vi "fpga_Fund FIFO Control.vi"(0 "Time stamp":fxp<+,64,32> format="%.42g", 1 "reset":bool, 2 "nominal frequency":enum16{"50 Hz", "60 Hz"}(ring), 5 "Frequency":fxp<+,32,8>, 7 "#ch":fxp<+,5,5>, 9 "PMU VI input valid":bool, 11 "PMU VI output valid":bool) -> (4 "Time Stamp out":fxp<+,64,32> format="%.42g", 8 "output frequency":T1 {"frequency timestamp [s]" format="%#.6g"})   [LabVIEW 2012, in "NI_EP_Protection_FPGA.lvlib"]
uses:
  <vilib>/addons/Electrical Power/Protection/NI_EP_Protection_FPGA.lvlib
  <vilib>/addons/Electrical Power/Protection/Protection Measurement/subVIs/fpga_OutputFrequency.ctl
  <vilib>/rvi/DataTransferAndStorage/Container/Common/niFpgaContainerMetaDataKey.ctl
  <vilib>/rvi/DataTransferAndStorage/Container/Common/niFpgaContainerState.ctl
  <vilib>/rvi/DataTransferAndStorage/Container/Common/niFpgaDataTypeControl.ctl
  <vilib>/rvi/DataTransferAndStorage/Container/Common/niFpgaContainerImplementationControl.ctl
  <vilib>/rvi/DataTransferAndStorage/Container/Common/niFpgaContainerArbitrationOptionsControl.ctl
  <vilib>/rvi/DataTransferAndStorage/Container/Common/niFpgaTransferTypeControl.ctl
  <vilib>/rvi/DataTransferAndStorage/Container/Common/niFpgaContainerInitializationParameters.ctl
  <vilib>/rvi/Memory/Memory_Types/niFpgaMemoryInterfaceConfiguration.ctl
  <vilib>/rvi/FIFO/Fifo_Types/niFpgaFifoControlLogicControl.ctl
  <vilib>/rvi/DataTransferAndStorage/Container/Common/niFpgaContainerGetUniqueNameForEmu.vi
  <vilib>/rvi/DataTransferAndStorage/Container/Common/niFpgaContainerSetEmuInfo.vi
  <vilib>/rvi/eio/common/nirviEmuReportErrorAndStop.vi
  <vilib>/rvi/Emulation/niFpgaSctlEmulationGetInTimedLoop.vi
  <vilib>/rvi/FIFO/Fifo_Resource/nirvififoEmulationSetSize.vi
  <vilib>/rvi/Emulation/niFpgaSctlEmulationFifoFullMgr.vi
  <vilib>/rvi/errors/niFpgaSetErrorForExecOnDevCompSimple.vi
  <vilib>/rvi/Emulation/niFpgaSctlEmulationResourceMgr.vi
  <vilib>/rvi/LocalResourceManager/LocalResourceManager.xnode
  <vilib>/rvi/DataTransferAndStorage/Container/XNode/niFpgaContainer.xnode
  <vilib>/rvi/FIFO/Fifo_Resource/nirvififoEmulationRead.vi
  <vilib>/rvi/FXPMathLib/basic elements/FxpDiscreteDelay/XNode/nifxpmath_DiscreteDelay.xnode
  <vilib>/rvi/FXPMathLib/FxpSub/XNode/nifxpmath_Sub.xnode
  <vilib>/rvi/FIFO/Fifo_Resource/nirvififoEmulationWrite.vi
  <vilib>/addons/Electrical Power/PQ/Resampling/NI_EP_Resample_FPGA.lvlib
  <vilib>/rvi/FXPMathLib/sim/FxpSim.dll
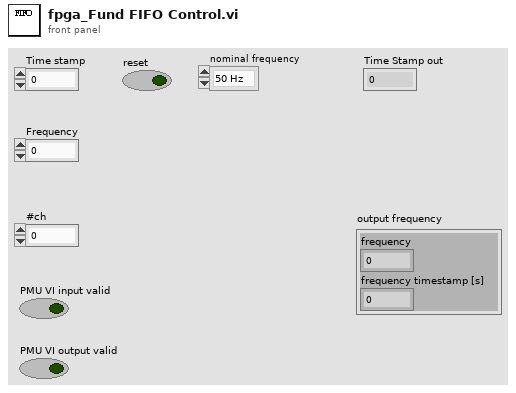
[diagram p1: front panel]
types:
  T1 = typedef "NI_EP_Protection_FPGA.lvlib/fpga_OutputFrequency.ctl" = cluster{"frequency":fxp<+,32,8>, "frequency timestamp [s]":fxp<+,64,32>}
  T2 = cluster{"frequency":fxp<+,32,8>, "frequency timestamp [s]":fxp<+,64,32>}
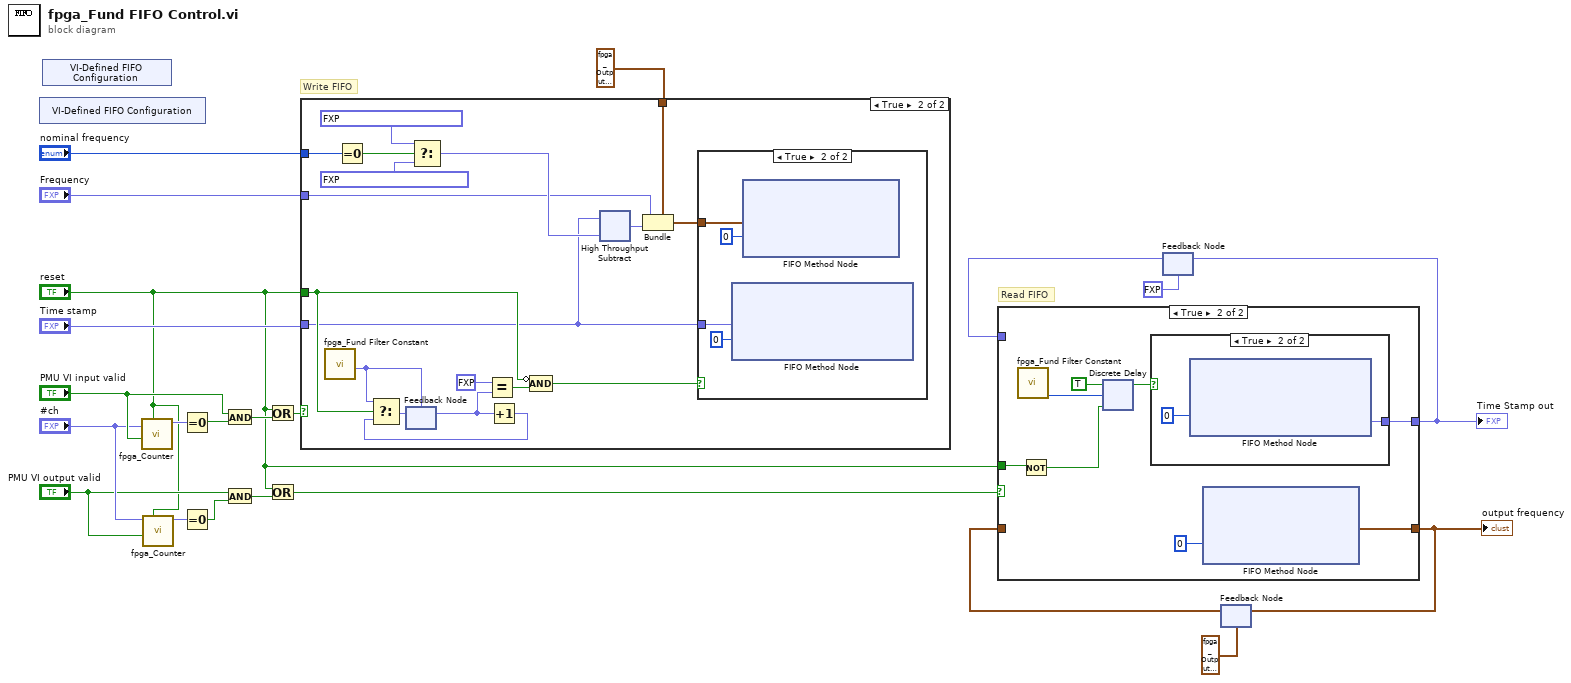
[diagram p0: block diagram]
diagram:
  # "Read FIFO"
  # "Write FIFO"
  n1 = xnode "VI-Defined FIFO Configuration"() -> ()  [unwired: 1 out]
  n2 = xnode "VI-Defined FIFO Configuration"() -> ()  [unwired: 1 out]
  n3 = call <vilib>:"fpga_Counter.vi"("reset"="reset", "Input Valid?"="PMU VI input valid", "upper limit"="#ch") -> ("count"=w10:fxp<+,5,5>)  [unwired: 7 in, 1 out]
  n4 = call <vilib>:"fpga_Counter.vi"("reset"="reset", "Input Valid?"="PMU VI output valid", "upper limit"="#ch") -> ("count"=w9:fxp<+,5,5>)  [unwired: 7 in, 1 out]
  n5 = Equal To 0?(x=w10) -> (x = 0?=w21:bool)
  n6 = Equal To 0?(x=w9) -> (x = 0?=w16:bool)
  n7 = And(x="PMU VI input valid", y=w21) -> (x .and. y?=w14:bool)
  n8 = And(x="PMU VI output valid", y=w16) -> (x .and. y?=w20:bool)
  n9 = Or(x="reset", y=w14) -> (x .or. y?=w13:bool)
  n10 = Or(x="reset", y=w20) -> (x .or. y?=w19:bool)
  n11 = case shown="True" w13 {
    tunnel: "Time stamp" -> [_ w25]
    tunnel: "reset" -> [_ w35]
    tunnel: "Frequency" -> [_ w24]
    tunnel: T1 {"frequency"=0.0, "frequency timestamp [s]"=0.0} ("output frequency") -> [_ w31]
    tunnel: "nominal frequency" -> [_ w30]
    frame False {
    }
    frame True {
      n12 = call <vilib>:"fpga_Fund Filter Constant.vi"() -> ("Start"=w34:fxp<+/-,4,4>)  [unwired: 8 in, 3 out]
      n13 = Equal To 0?(x=w30) -> (x = 0?=w29:bool)
      n14 = feedback #1(w34) -> (w38:fxp<+/-,4,4>)
      n15 = Select(t=fxp<+,18,-4> 0.060719966888427734 ("y"), s=w29, f=fxp<+,18,-4> 0.05672001838684082 ("y")) -> (s? t:f=w27:fxp<+,18,-4>)
      n16 = Equal?(x=fxp<+/-,4,4> 4.0, y=w38) -> (x = y?=w36:bool)
      n17 = Increment(x=w38) -> (x+1=w39:fxp<+,3,3>)
      n18 = Select(t=w34, s=w35, f=w39) -> (s? t:f=w40:fxp<+/-,4,4>)
      n19 = feedback-in #1(w40) -> ()
      n20 = Compound Arithmetic op=AND(invert w35, w36) -> (w33:bool)
      n21 = xnode "High Throughput Subtract"("x"=w25, "y"=w27) -> ("x-y"=w32:fxp<+,64,32>)
      n22 = Bundle(cluster=w31, "frequency"=w24, "frequency timestamp [s]"=w32) -> (w23:T1)
      n23 = case shown="True" w33 {
        tunnel: w25 -> [_ w43]
        tunnel: w23 -> [_ w41]
        frame False {
        }
        frame True {
          n24 = xnode ("FIFO Method Node")("Element"=w43, "Timeout"=0) -> ()  [unwired: 1 in, 2 out]
          n25 = xnode ("FIFO Method Node")("Element"=w41, "Timeout"=0) -> ()  [unwired: 1 in, 2 out]
        }
      }
    }
  }
  n26 = feedback #2(fxp<+,64,32> 0.0 ("Element")) -> (w17:fxp<+,64,32>)
  n27 = feedback #3(T1 {"frequency"=0.0, "frequency timestamp [s]"=0.0} ("output frequency")) -> (w1:T1)
  n28 = case shown="True" w19 {
    tunnel: "reset" -> [_ w53]
    tunnel: [w46 w54] -> w18
    tunnel: w17 -> [w46 _]
    tunnel: [w45 w47] -> w3
    tunnel: w1 -> [w45 _]
    frame False {
    }
    frame True {
      n29 = call <vilib>:"fpga_Fund Filter Constant.vi"() -> ("Total Delay"=w49:u8)  [unwired: 8 in, 3 out]
      n30 = Not(x=w53) -> (.not. x?=w51:bool)
      n31 = xnode "Discrete Delay"("D"=TRUE, "n-1[0..31]"=w49, "enable"=w51) -> ("Q"=w50:bool)
      n32 = case shown="True" w50 {
        tunnel: [_ w55] -> w54
        frame False {
        }
        frame True {
          n33 = xnode ("FIFO Method Node")("Timeout"=0) -> ("Element"=w55:fxp<+,64,32>)  [unwired: 1 in, 2 out]
        }
      }
      n34 = xnode ("FIFO Method Node")("Timeout"=0) -> ("Element"=w47:T2)  [unwired: 1 in, 2 out]
    }
  }
  "Time Stamp out" <- w18
  "output frequency" <- w3
  n35 = feedback-in #2(w18) -> ()
  n36 = feedback-in #3(w3) -> ()
